vi "Update.vi"(8 "error in (no error)":errorcluster, 10 "Engine in":refnum<class "Engine.lvclass">, 11 "BounceDemo in":refnum<class "BounceDemo.lvclass">) -> (0 "error out":errorcluster, 2 "Engine out":refnum<class "Engine.lvclass">, 3 "BounceDemo out":refnum<class "BounceDemo.lvclass">)   [LabVIEW 2019, in "RT_Game.lvlib" / "BounceDemo.lvclass"]
uses:
  BounceDemo.lvclass
  C:/Users/FreshBob/Dropbox/VIs/myRIO_GameConsole/RT/RT_Game/Game/Game.lvclass
  C:/Users/FreshBob/Dropbox/VIs/myRIO_GameConsole/RT/RT_Game/Bouncer/Bouncer.lvclass
  Engine/Engine.lvclass
  Menu/States.ctl
  Game/Game.lvclass/Game.ctl
  Bouncer/Bouncer.lvclass/Bouncer.ctl
  BounceDemo.lvclass/BounceDemo.ctl
  AttractScreen/AttractScreen.lvclass
  Engine/Engine.lvclass/Engine.ctl
  Engine/Write NextGame.vi
  Engine/Write SwitchGame_.vi
  Game/Read State.vi
  Bouncer/Read level.vi
  Bouncer/Bouncer.lvclass
  Game/Game.lvclass
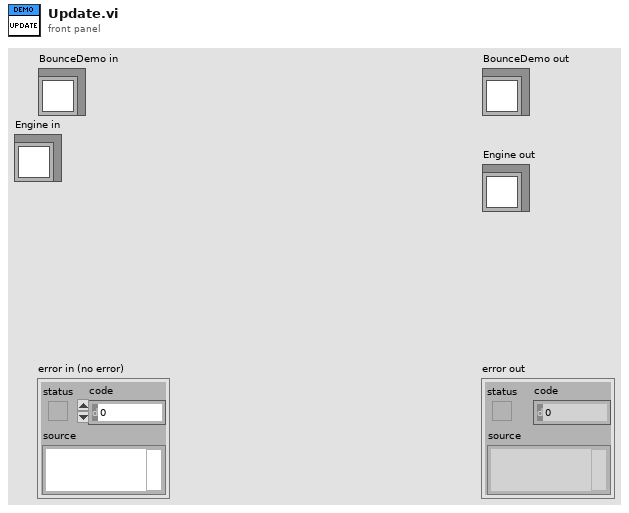
[diagram p1: front panel]
types:
  T1 = typedef "RT_Game.lvlib/Game.lvclass/States.ctl" = enum16{"Init", "Restart", "Menu", "Game", "Resume", "ToggleSingleplayer", "LoadNextGame", "ExitToMenu", "NewHighscore", "GameOver", "SlideOut", "FadeToMenu", "StartFadeToMenu"}
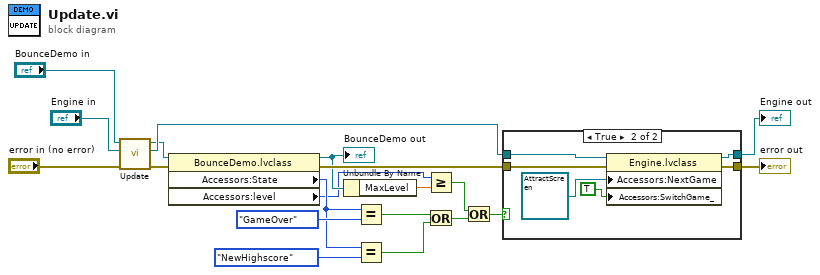
[diagram p0: block diagram]
diagram:
  n1 = call-parent "Update.vi"("error in (no error)"="error in (no error)", "Engine in"="Engine in", "Bouncer in"="BounceDemo in") -> ("error out"=w20:errorcluster, "Engine out"=w15:refnum<class "Engine.lvclass">, "Bouncer out"=w12:refnum<class "BounceDemo.lvclass">)  [unwired: 6 in]
  n2 = property class="BounceDemo.lvclass"(reference=w12, error in=w20) -> (reference out=w11:refnum<class "BounceDemo.lvclass">, error out=w13:errorcluster, "Accessors:State"=w8:T1, "Accessors:level"=w3:i16)
  "BounceDemo out" <- w11
  n3 = Unbundle By Name(w11) -> ("MaxLevel"=w2:dbl)
  n4 = Equal?(x=w8, y=States."GameOver") -> (x = y?=w5:bool)
  n5 = Equal?(x=w8, y=States."NewHighscore") -> (x = y?=w4:bool)
  n6 = Greater Or Equal?(x=w3, y=w2) -> (x >= y?=w1:bool)
  n7 = Or(x=w5, y=w4) -> (x .or. y?=w6:bool)
  n8 = Or(x=w1, y=w6) -> (x .or. y?=w7:bool)
  n9 = case shown="True" w7 {
    tunnel: w13 -> [w21 w28]
    tunnel: [w21 w27] -> w16
    tunnel: w15 -> [w22 w26]
    tunnel: [w22 w25] -> w14
    frame False {
    }
    frame True {
      n10 = property class="Engine.lvclass"(reference=w26, error in=w28, "Accessors:NextGame"=refnum<class "AttractScreen.lvclass"> refnum ("RT_Game.lvlib:AttractScreen.lvclass"), "Accessors:SwitchGame_"=TRUE ("SwitchGame_")) -> (reference out=w25:refnum<class "Engine.lvclass">, error out=w27:errorcluster)
    }
  }
  "error out" <- w16
  "Engine out" <- w14
